vi "Timestamp to ISO8601 Ordinal Date.vi"(9 "UTC? (F)":bool, 11 "Timestamp (now)":timestamp) -> (3 "ISO8601 Ordinal Date":string)   [LabVIEW 2013]
uses:
  formatter.iso8601/DateTime.ISO8601.lvclass
  formatter.iso8601/ISO8601 Date Formats.ctl
  formatter.iso8601/DateTime.ISO8601.lvclass/DateTime.ISO8601.ctl
  epoch/Epoch.lvclass
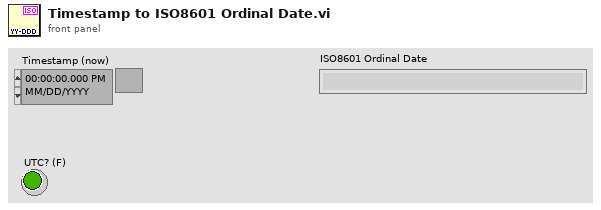
[diagram p1: front panel]
types:
  T1 = typedef "DateTime.ISO8601.lvclass/ISO8601 Date Formats.ctl" = enum16{"UTC Date-Time", "Date", "Week", "Week-Day", "Month-Day", "Ordinal Date"}
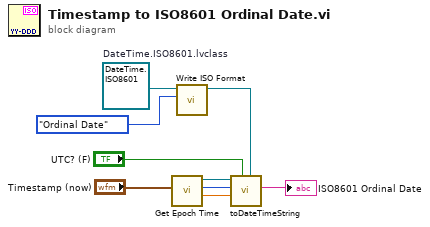
[diagram p0: block diagram]
diagram:
  w9 = refnum<class "DateTime.ISO8601.lvclass"> refnum  # DateTime.ISO8601.lvclass
  n1 = call "Get Epoch Time.vi"("Timestamp (now)"="Timestamp (now)") -> ("Fractional Second"=w4:dbl, "Epoch Time (s)"=w5:i64, "Epoch out"=w6:refnum<class "Epoch.lvclass">)  [unwired: 8 in]
  n2 = call "Write ISO Format.vi"("ISO Format"=ISO8601_Date_Formats."Ordinal Date", "DateTime.ISO8601 in"=w9) -> ("DateTime.ISO8601 out"=w7:refnum<class "DateTime.ISO8601.lvclass">)  [unwired: 9 in]
  n3 = call "toDateTimeString.vi"("DateTimeFormatter (ISO8601)"=w7, "UTC? (F)"="UTC? (F)", "Fractional Second"=w4, "Epoch Time (s)"=w5, "Epoch"=w6) -> ("DateTime string"=→"ISO8601 Ordinal Date":string)  [unwired: 4 in, 2 out]
